vi "ex2.vi"   [LabVIEW 2022 SP3]
uses:
  <vilib>/numeric/Random Number (Range) DBL.vi
types:
  T1 = enum16{"open", "replace", "create", "open or create", "replace or create", "replace or create with confirmation"}
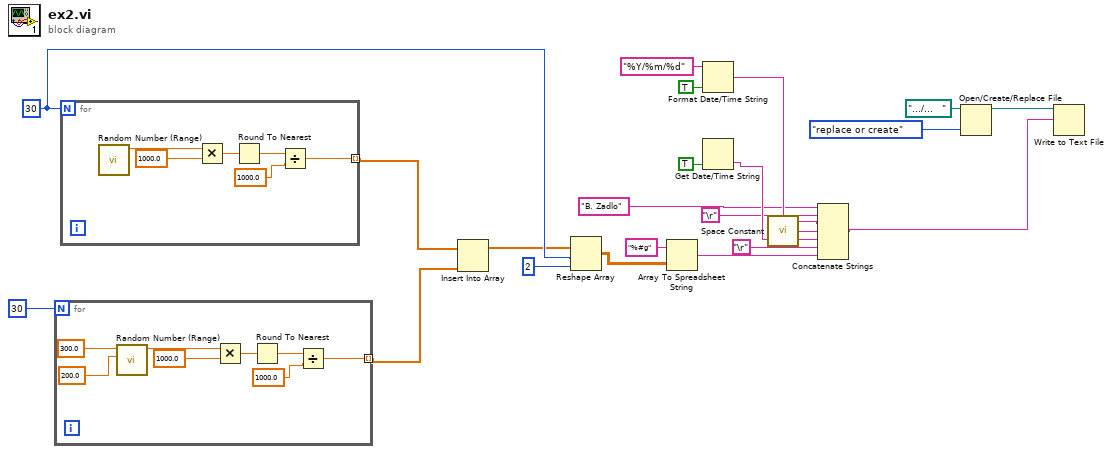
[diagram p0: block diagram]
diagram:
  w19 = 30
  n1 = for {
    N: 30 -> [_]
    tunnel: [w25] -> w20 mode=indexing
    n2 = call-poly <vilib>:"Random Number (Range).vi"("lower bound (0)"=200.0, "upper bound (100)"=300.0) -> ("number"=w29:dbl)  [unwired: 9 in]
    n3 = Multiply(x=w29, y=1000.0) -> (x*y=w28:dbl)
    n4 = Round To Nearest(number=w28) -> (nearest integer value=w27:dbl)
    n5 = Divide(x=w27, y=1000.0) -> (x/y=w25:dbl)
  }
  n6 = for {
    N: w19 -> [_]
    tunnel: [w31] -> w21 mode=indexing
    n7 = call-poly <vilib>:"Random Number (Range).vi"() -> ("number"=w35:dbl)  [unwired: 11 in]
    n8 = Multiply(x=w35, y=1000.0) -> (x*y=w34:dbl)
    n9 = Round To Nearest(number=w34) -> (nearest integer value=w33:dbl)
    n10 = Divide(x=w33, y=1000.0) -> (x/y=w31:dbl)
  }
  n11 = Insert Into Array(array=w21, new element=w20) -> (w17:dbl[])  [unwired: 1 in]
  n12 = Reshape Array(w17, w19, 2 ("dimension size")) -> (w15:dbl[][])
  n13 = Array To Spreadsheet String(array=w15, 3:"%#g" ("format string")) -> (spreadsheet string=w14:string)  [unwired: 1 in]
  n14 = Format Date/Time String(time format string (%c)="%Y/%m/%d", UTC format=TRUE) -> (date/time string=w7:string)  [unwired: 1 in]
  n15 = Get Date/Time String(want seconds? (F)=TRUE) -> (time string=w11:string)  [unwired: 2 in, 1 out]
  n16 = call <vilib>:"Space Constant.vi"() -> ("String"=w10:string)
  n17 = Concatenate Strings("B. Zadlo" ("string"), "\r", w7, w10, w11, "\r", w14) -> (w1:string)
  n18 = Open/Create/Replace File(file path (use dialog)=path ".../...   ", operation (0:open)=T1."replace or create") -> (refnum out=w2:refnum<file>)  [unwired: 4 in, 2 out]
  n19 = Write to Text File(file (use dialog)=w2, text=w1) -> ()  [unwired: 2 in, 3 out]
